vi "WILT Clean Up Agilent Entries.vi"(11 "Agilent Channels Raw":T1[](array[typedef])) -> (3 "Full Agilent Array":T1[](array[typedef]))   [LabVIEW 2016]
uses:
  Type Definitions/WILT Agilent Channel Definition.ctl
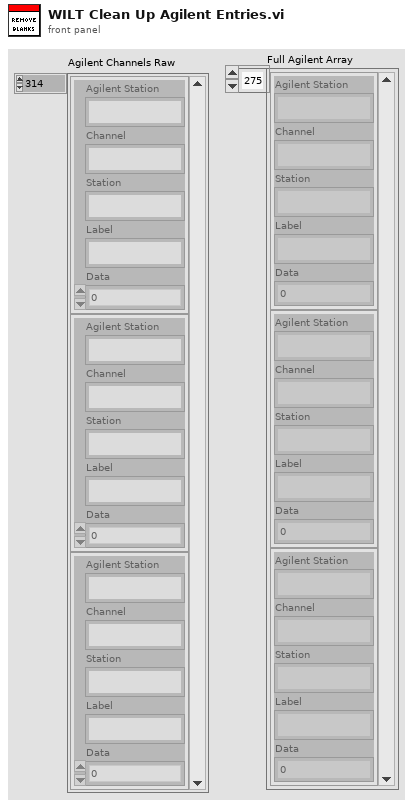
[diagram p1: front panel]
types:
  T1 = typedef "WILT Agilent Channel Definition.ctl" = cluster{"Channel":string, "Station":string, "Label":string, "Agilent Station":string, "Data":dbl}
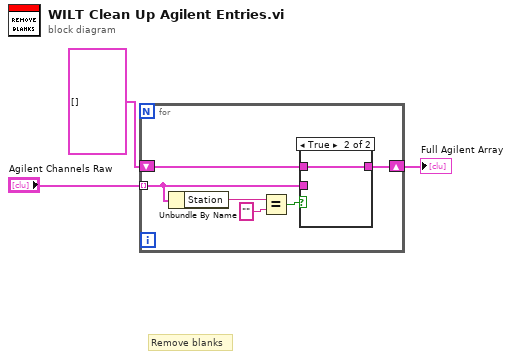
[diagram p0: block diagram]
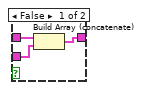
[diagram p2: hidden frame]
diagram:
  # "Remove blanks"
  n1 = for {
    tunnel: "Agilent Channels Raw" -> [w9] mode=indexing
    shift-right: [w8] -> w3
    shift-left: T1[] [] -> [w7]
    n2 = Unbundle By Name(w9) -> ("Station"=w4:string)
    n3 = Equal?(x=w4, y="") -> (x = y?=w5:bool)
    n4 = case shown="True" w5 {
      tunnel: w9 -> [w12 _]
      tunnel: w7 -> [w11 w13]
      tunnel: [w10 w13] -> w8
      frame False {
        n5 = Build Array (concatenate)(w11, w12) -> (w10:T1[])
      }
      frame True {
      }
    }
  }
  "Full Agilent Array" <- w3
